vi "Мультиплексор(2 одноразрядных операнда).vi"(1 "c":bool, 2 "y":bool, 3 "x":bool) -> (0 "r":bool)   [LabVIEW 2013]
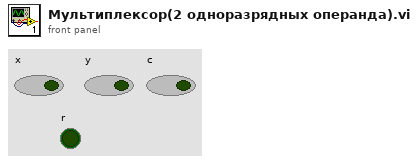
[diagram p1: front panel]
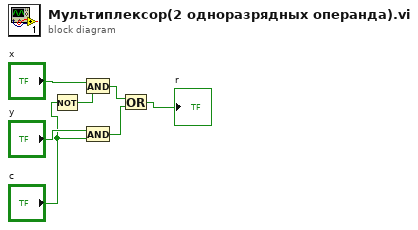
[diagram p0: block diagram]
diagram:
  n1 = Not(x="c") -> (.not. x?=w4:bool)
  n2 = And(x="x", y=w4) -> (x .and. y?=w3:bool)
  n3 = And(x="y", y="c") -> (x .and. y?=w2:bool)
  n4 = Or(x=w3, y=w2) -> (x .or. y?=→"r":bool)
